vi "Set Lockin IV Mode.vi"(8 "error in (no error)":errorcluster, 10 "IV Mode?":bool, 11 "MeasurementSMO in":refnum<class "AFM_Litho_Plugin.IV.lvclass">) -> (0 "error out":errorcluster, 3 "MeasurementSMO out":refnum<class "AFM_Litho_Plugin.IV.lvclass">)   [LabVIEW 2019, in "AFM_Litho_Plugin.IV.lvclass"]
uses:
  AFM_Litho_Plugin.IV.lvclass
  AFM_Litho_Plugin.IV.lvclass/AFM_Litho_Plugin.IV.ctl
  1b863cf5-8067-4920-aeba-5c929888f10a.vi
  1b863cf5-8067-4920-aeba-5c929888f10a.vi/ff40df25-0e41-4205-825d-56c19dc320b6.vi
  <vilib>/Utility/Debug Log/Display.vi
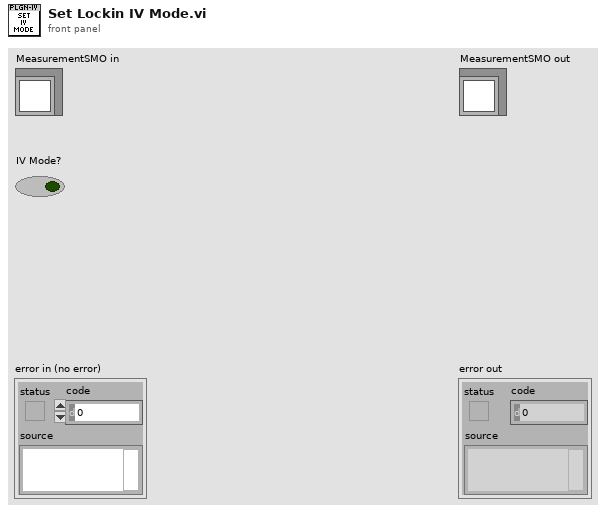
[diagram p1: front panel]
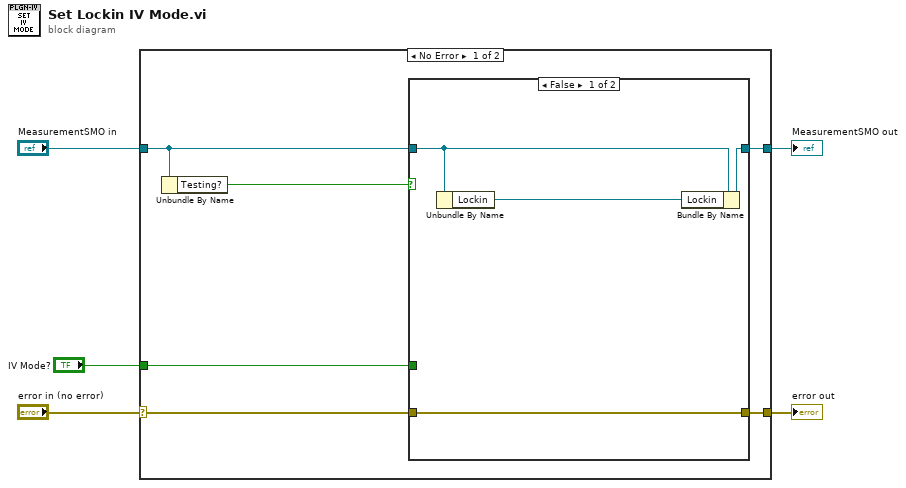
[diagram p0: block diagram]
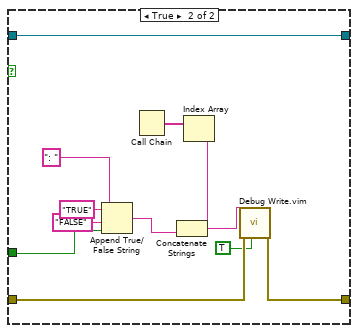
[diagram p2: hidden frame]
diagram:
  n1 = case shown="No Error" "error in (no error)" {
    selector: "error in (no error)" -> [w7 w29]
    tunnel: [w8 w29] -> w4
    tunnel: [w9 w28] -> w2
    tunnel: "MeasurementSMO in" -> [w10 w28]
    tunnel: "IV Mode?" -> [w6 _]
    frame No Error {
      n2 = Unbundle By Name(w10) -> ("Testing?"=w11:bool)
      n3 = case shown="False" w11 {
        tunnel: w10 -> [w14 w27]
        tunnel: [w15 w27] -> w9
        tunnel: [w12 w18] -> w8
        tunnel: w7 -> [w12 w17]
        tunnel: w6 -> [_ w24]
        frame False {
          n4 = Unbundle By Name(w14) -> ("Lockin"=w13:refnum<class "Instrument.Lockin.lvclass">)
          n5 = Bundle By Name(cluster=w14, "Lockin"=w13) -> (w15:refnum<class "AFM_Litho_Plugin.IV.lvclass">)
        }
        frame True {
          n6 = Append True/False String(1:w24, 2:"FALSE" ("false string"), 3:"TRUE" ("true string"), 4:": " ("string (\"\")")) -> (0:w21:string)
          n7 = Call Chain() -> (call chain=w23:string[])
          n8 = Index Array(array=w23) -> (element=w20:string)  [unwired: 1 in]
          n9 = Concatenate Strings(w20, w21) -> (w19:string)
          n10 = call "Debug Write.vim"("include timestamp? (F)"=TRUE, "error in (no error)"=w17, "value"=w19) -> ("error out"=w18:errorcluster)  [unwired: 8 in]
        }
      }
    }
    frame Error {
    }
  }
  "error out" <- w4
  "MeasurementSMO out" <- w2
